vi "pid2.vi"(7 "当前":dbl, 8 "kd":dbl, 9 "ki":dbl, 10 "kp":dbl, 11 "目标":dbl) -> (2 "out":dbl)   [LabVIEW 2022 SP3]
panel:
  out "d":dbl
  out "p":dbl
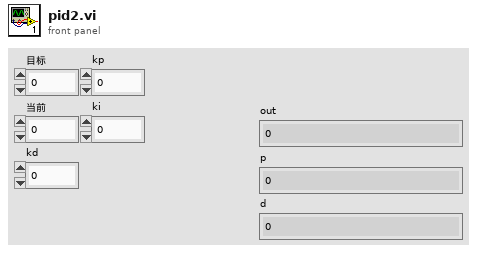
[diagram p1: front panel]
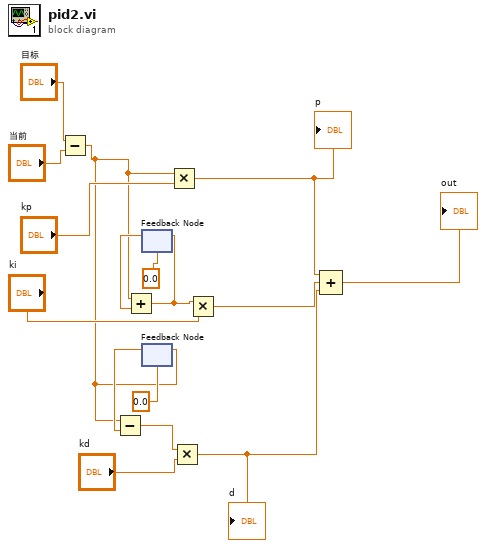
[diagram p0: block diagram]
diagram:
  n1 = Subtract(x="目标", y="当前") -> (x-y=w1:dbl)
  n2 = feedback #1(0.0) -> (w13:dbl)
  n3 = Add(x=w1, y=w13) -> (x+y=w11:dbl)
  n4 = feedback-in #1(w11) -> ()
  n5 = feedback #2(0.0) -> (w9:dbl)
  n6 = Subtract(x=w1, y=w9) -> (x-y=w7:dbl)
  n7 = feedback-in #2(w1) -> ()
  n8 = Multiply(x=w1, y="kp") -> (x*y=w5:dbl)
  "p" <- w5
  n9 = Multiply(x=w7, y="kd") -> (x*y=w3:dbl)
  "d" <- w3
  n10 = Multiply(x=w11, y="ki") -> (x*y=w4:dbl)
  n11 = Compound Arithmetic op=ADD(w5, w4, w3) -> (→"out":dbl)
